vi "LV8_7.vi"() -> ()   [LabVIEW 2016]
uses:
  <vilib>/imath/engines/lvmath2/RunTimeEngine/BuiltInFunctions/randnormal/NIMS_randnormal(Str,I32).vi
  <vilib>/imathl/engines/lvmath/Functions/Error Handling/Create Error.vi
  <vilib>/imath/engines/lvmath2/RunTimeEngine/BuiltInFunctions/randnormal/NIMS_randnormal(1,I32).vi
  <vilib>/imath/engines/lvmath2/RunTimeEngine/ErrorHandling/NIMS_Error From Error Code.vi
  <vilib>/imath/engines/lvmath2/RunTimeEngine/BuiltInFunctions/linramp/NIMS_linramp.vi
  <vilib>/imath/engines/lvmath2/RunTimeEngine/ArithmeticOperatorToken/NIMS_ArithmeticOperator_plus.vi
  <instcachedir>/0/NIMS_ArithmeticOperator_plus_0120E0498A0F4B4B9BDCAC2554767A4E.lvgen/NIMS_ArithmeticOperator_plus_0120E0498A0F4B4B9BDCAC2554767A4E_004.vi
  <vilib>/imath/engines/lvmath2/RunTimeEngine/BuiltInFunctions/fft/NIMS_fft(GV).vi
  <instcachedir>/0/NIMS_fft(GV)_4C6467FC22F84E4BA42517A07EF978B0.lvgen/NIMS_fft(GV)_4C6467FC22F84E4BA42517A07EF978B0_000.vi
  <vilib>/imath/engines/lvmath2/RunTimeEngine/BuiltInFunctions/abs/NIMS_abs(signed).vi
  <instcachedir>/0/NIMS_abs(signed)_C4FCB8E6058B49B797C7C8D53CA5F6EC.lvgen/NIMS_abs(signed)_C4FCB8E6058B49B797C7C8D53CA5F6EC_006.vi
  <vilib>/imath/engines/lvmath2/RunTimeEngine/BuiltInFunctions/findnz/NIMS_[1o]_findnz(GRowV).vi
  <instcachedir>/0/NIMS_[1o]_findnz(GRowV)_1AF74843B4874134ADE908C0A4A72F3C.lvgen/NIMS_[1o]_findnz(GRowV)_1AF74843B4874134ADE908C0A4A72F3C_000.vi
  <vilib>/imath/engines/lvmath2/RunTimeEngine/IndexReplace/NIMS V(V)=S.vi
  <instcachedir>/0/NIMS V(V)=S_4469BB7E0DD5440190F262393D16598E.lvgen/NIMS V(V)=S_4469BB7E0DD5440190F262393D16598E_002.vi
  <vilib>/imath/engines/lvmath2/RunTimeEngine/BuiltInFunctions/ifft/NIMS_ifft(CV).vi
  <vilib>/imath/engines/lvmath2/RunTimeEngine/ArithmeticOperatorToken/NIMS_ArithmeticOperator_times.vi
  <instcachedir>/0/NIMS_ArithmeticOperator_times_953B34F74CAC448FB707D816A29CC5F0.lvgen/NIMS_ArithmeticOperator_times_953B34F74CAC448FB707D816A29CC5F0_000.vi
  <vilib>/imath/engines/lvmath2/RunTimeEngine/BuiltInFunctions/sum/NIMS_sum(GV).vi
  <instcachedir>/0/NIMS_sum(GV)_67F5EC36BC034E54A6BEC5B0673C00E5.lvgen/NIMS_sum(GV)_67F5EC36BC034E54A6BEC5B0673C00E5_000.vi
  <vilib>/imath/engines/lvmath2/RunTimeEngine/ErrorHandling/NIMS_Create Error From Enums.vi
  <vilib>/imath/engines/lvmath2/RunTimeEngine/NodeEndStatement/NIMS_NodeEndStatement_Output.vi
  <instcachedir>/0/NIMS_NodeEndStatement_Output_53EC0D466D134D7ABD903AC30B43404B.lvgen/NIMS_NodeEndStatement_Output_53EC0D466D134D7ABD903AC30B43404B_009.vi
  <instcachedir>/0/NIMS_NodeEndStatement_Output_53EC0D466D134D7ABD903AC30B43404B.lvgen/NIMS_NodeEndStatement_Output_53EC0D466D134D7ABD903AC30B43404B_005.vi
  <instcachedir>/0/NIMS_NodeEndStatement_Output_53EC0D466D134D7ABD903AC30B43404B.lvgen/NIMS_NodeEndStatement_Output_53EC0D466D134D7ABD903AC30B43404B_004.vi
  <vilib>/imath/engines/lvmath2/RunTimeEngine/ErrorHandling/NIMS_Finalize Error.vi
panel:
  out "SNR (dB)":dbl=3.669052525118055
  in  "noise level":dbl(slide)=5.0 scale=0.1..15.0
  in  "threshold":dbl(slide)=0.9 scale=0.01..1.0
  in  "f2":dbl(slide)=200.0 scale=100.0..300.0
  in  "f1":dbl(slide)=125.0 scale=100.0..300.0
  out "Filtered signal (frequency domain)":cluster{"W":i32[], "FY":dbl[]}(graph)
  out "Filtered signal (time domain)":cluster{"N":dbl[], "X":dbl[]}(graph)
  out "Noisy signal (frequency domain)":cluster{"W":dbl[], "FYI":dbl[]}[](graph)=[{"W"=array[1000 elements], "FYI"=array[1000 elements]}, {"W"=[0.0, 999.0], "FYI"=[1.8, 1.8]}]
  out "Noisy signal (time domain)":cluster{"N":dbl[], "Y":dbl[]}(graph)
  in  "stop":bool
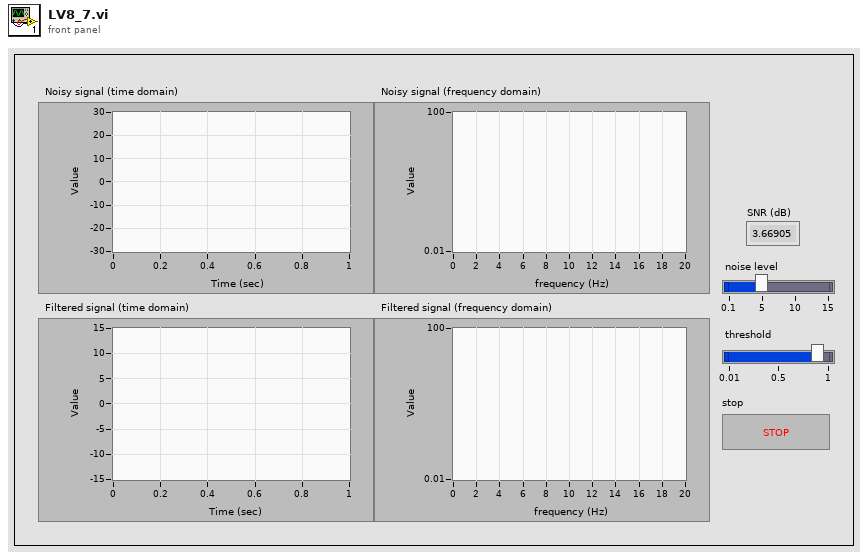
[diagram p1: front panel]
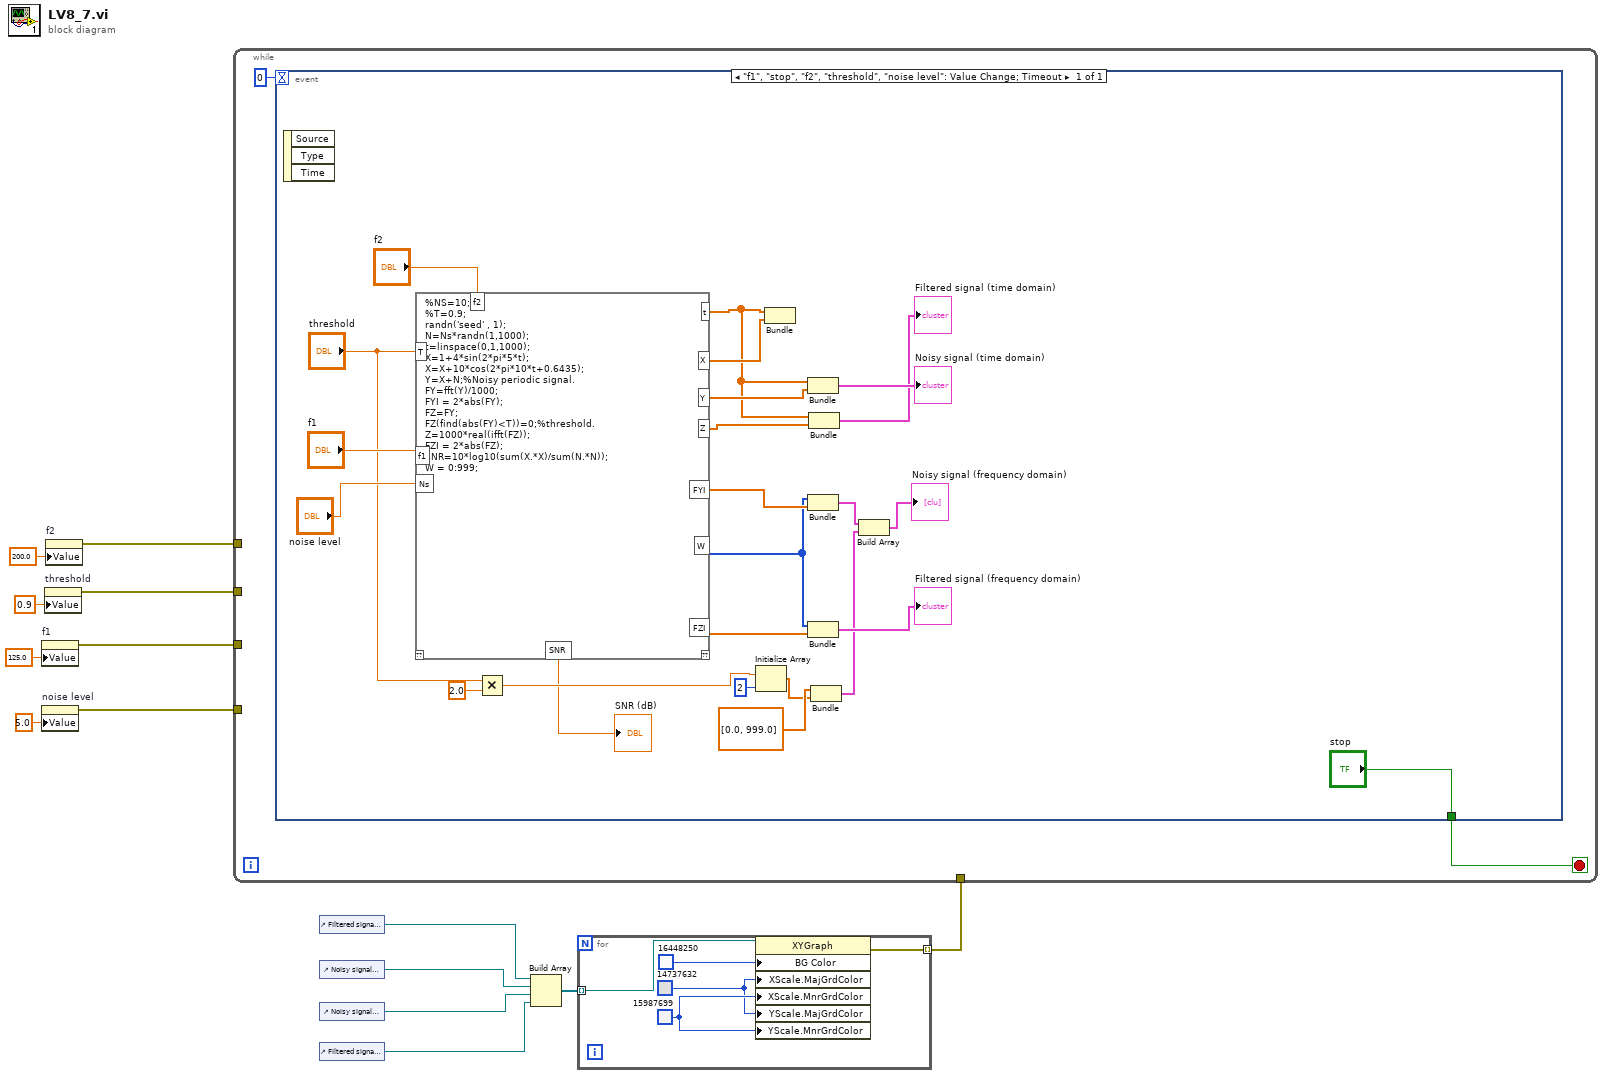
[diagram p0: block diagram]
diagram:
  n1 = property on="f1" class="Slide (strict)"("Value"=125.0 ("Interference level")) -> (error out=w12:errorcluster)  [unwired: 2 in, 1 out]
  n2 = property on="noise level" class="Slide (strict)"("Value"=5.0 ("notch frequency")) -> (error out=w8:errorcluster)  [unwired: 2 in, 1 out]
  n3 = property on="threshold" class="Slide (strict)"("Value"=0.9 ("pole radius")) -> (error out=w13:errorcluster)  [unwired: 2 in, 1 out]
  n4 = property on="f2" class="Slide (strict)"("Value"=200.0 ("Interference frequency")) -> (error out=w14:errorcluster)  [unwired: 2 in, 1 out]
  n5 = control-ref of="Filtered signal (time domain)"() -> (w5:refnum<vi>)
  n6 = control-ref of="Noisy signal (time domain)"() -> (w4:refnum<vi>)
  n7 = control-ref of="Noisy signal (frequency domain)"() -> (w3:refnum<vi>)
  n8 = control-ref of="Filtered signal (frequency domain)"() -> (w2:refnum<vi>)
  n9 = Build Array(w5, w4, w3, w2) -> (w6:refnum<vi>[])
  n10 = for {
    tunnel: w6 -> [w16] mode=indexing
    tunnel: [w15] -> w1 mode=indexing
    w18 = u32 15987699
    w17 = u32 14737632
    n11 = property class="XYGraph"(reference=w16, "BG Color"=u32 16448250, "XScale.MajGrdColor"=w17, "XScale.MnrGrdColor"=w18, "YScale.MajGrdColor"=w17, "YScale.MnrGrdColor"=w18) -> (error out=w15:errorcluster)  [unwired: 1 in, 1 out]
  }
  n12 = while {
    tunnel: w14 -> [_]
    tunnel: w13 -> [_]
    tunnel: w12 -> [_]
    tunnel: w8 -> [_]
    tunnel: w1 -> [_]
    stop <- w21 stop-if-true
    n13 = event shown="[0] \"f1\", \"stop\", \"f2\", \"threshold\", \"noise level\": Value Change;  Timeout" {
      selector: _ -> [_]
      dyn-events: _ -> [_]
      timeout: 0 -> [_]
      tunnel: ["stop"] -> w21
      event "f1", "stop", "f2", "threshold", "noise level": Value Change; Timeout {
        n14 = event-data() -> ()  [unwired: 1 in, 3 out]
        n15 = mathscript code="%NS=10;\n%T=0.9;\nrandn('seed' , 1);\nN=Ns*randn(1,1000);\nt=linspace(0,1,1000);\nX=1+4*sin(2*pi*5*t);\nX=X+10*cos(2*pi*10*t+0.6435);\nY=X+N;%Noisy periodic signal.\nFY=fft(Y)/1000;\nFYI = 2*abs(FY);\nFZ=FY;\nFZ(find(abs(FY)<T))=0;%threshold.\nZ=1000*real(ifft(FZ)); \nFZI = 2*abs(FZ);\nSNR=10*log10(sum(X.*X)/sum(N.*N));\nW = 0:999;"("T"="threshold", "f1"="f1", "f2"="f2", "Ns"="noise level") -> ("Y"=w43:dbl[], "X"=w44:dbl[], "W"=w39:i32[], "FZI"=w41:dbl[], "t"=w33:dbl[], "FYI"=w40:dbl[], "Z"=w34:dbl[], "SNR"=→"SNR (dB)":cdb)  [unwired: 1 in, 1 out]
        n16 = Multiply(x="threshold", y=2.0) -> (x*y=w24:dbl)
        n17 = Initialize Array(w24, 2 ("dimension size")) -> (w26:dbl[])
        n18 = Bundle("t"=w33, "X"=w44) -> ()  [unwired: 1 in, 1 out]
        n19 = Bundle("t"=w33, "Y"=w43) -> (→"Noisy signal (time domain)":cluster{"t":dbl[], "Y":dbl[]})  [unwired: 1 in]
        n20 = Bundle("W"=w39, "FYI"=w40) -> (w30:cluster{"W":i32[], "FYI":dbl[]})  [unwired: 1 in]
        n21 = Bundle("W"=w39, "FZI"=w41) -> (→"Filtered signal (frequency domain)":cluster{"W":i32[], "FZI":dbl[]})  [unwired: 1 in]
        n22 = Bundle("t"=w33, "Z"=w34) -> (→"Filtered signal (time domain)":cluster{"t":dbl[], "Z":dbl[]})  [unwired: 1 in]
        n23 = Bundle(dbl[] [0.0, 999.0], w26) -> (w29:cluster{dbl[], dbl[]})  [unwired: 1 in]
        n24 = Build Array(w30, w29) -> (→"Noisy signal (frequency domain)":cluster{"W":dbl[], "FYI":dbl[]}[])
      }
    }
  }
